vi "Merge in DB.vi"(0 "DBMap in":refnum<class "DBMap.lvclass">, 5 "SQLite DB Path":path, 11 "error in (no error)":errorcluster {"code" format="Error %.0f"}) -> (4 "DBMap out":refnum<class "DBMap.lvclass">, 15 "error out":errorcluster {"code" format="Error %.0f"})   [LabVIEW 2020, in "DBMap.lvclass"]
uses:
  DBMap.lvclass
  DBMap.lvclass/DBMap.ctl
  <vilib>/drjdpowell/SQLite Library/SQL Statement/SQL Statement.lvclass/SQL Statement.ctl
  <vilib>/drjdpowell/SQLite Library/SQL Connection/Connection.lvclass
  <vilib>/drjdpowell/SQLite Library/SQL Statement/SQL Statement.lvclass
  <vilib>/drjdpowell/SQLite Library/Transaction Helpers/Transaction.lvlib
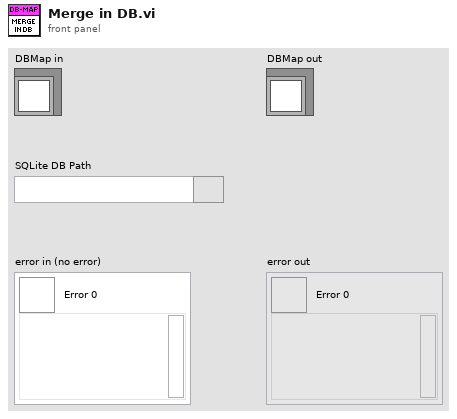
[diagram p1: front panel]
types:
  T1 = typedef "Semaphore RefNum" = refnum<k1>
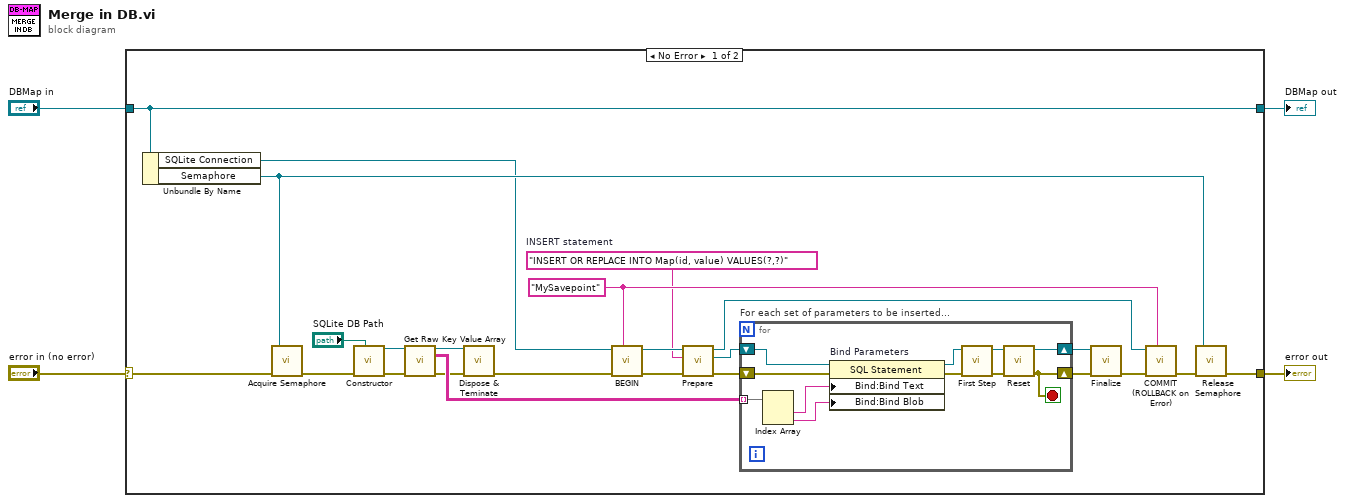
[diagram p0: block diagram]
diagram:
  n1 = case shown="No Error" "error in (no error)" {
    selector: "error in (no error)" -> [w27 w41]
    tunnel: [w26 w41] -> w3
    tunnel: [w28 w40] -> w1
    tunnel: "DBMap in" -> [w28 w40]
    frame No Error {
      w20 = "MySavepoint" ("Savepoint name")
      w15 = "INSERT OR REPLACE INTO Map(id, value) VALUES(?,?)"  # INSERT statement
      n2 = Unbundle By Name(w28) -> ("SQLite Connection"=w8:refnum<class "Connection.lvclass">, "Semaphore"=w25:T1)
      n3 = call <vilib>:"Acquire Semaphore.vi"("error in (no error)"=w27, "semaphore"=w25) -> ("error out"=w24:errorcluster)  [unwired: 3 in, 2 out]
      n4 = call "Constructor.vi"("SQLite DB Path"="SQLite DB Path", "error in (no error)"=w24) -> ("error out"=w11:errorcluster, "DBMap out"=w10:refnum<class "DBMap.lvclass">)  [unwired: 8 in]
      n5 = call "Get Raw Key Value Array.vi"("DBMap in"=w10, "error in (no error)"=w11) -> ("DBMap out"=w5:refnum<class "DBMap.lvclass">, "KV Array Raw"=w9:string[][], "error out"=w7:errorcluster)  [unwired: 11 in]
      n6 = call-dynamic "Dispose & Teminate.vi"("DBMap in"=w5, "error in (no error)"=w7) -> ("error out"=w6:errorcluster)  [unwired: 12 in, 1 out]
      n7 = call <vilib>:"BEGIN.vi"("Savepoint name"=w20, "error in (no error)"=w6, "SQLite Connection in"=w8) -> ("error out"=w19:errorcluster, "SQLite Connection"=w18:refnum<class "Connection.lvclass">)  [unwired: 7 in]
      n8 = call <vilib>:"Prepare.vi"("error in (no error)"=w19, "SQL"=w15, "SQLite Connection in"=w18) -> ("error out"=w14:errorcluster, "SQL Statement"=w13:refnum<class "SQL Statement.lvclass">, "SQLite Connection"=w21:refnum<class "Connection.lvclass">)  [unwired: 4 in, 2 out]
      n9 = for "For each set of parameters to be inserted..." {
        shift-right: [w33] -> w16
        shift-left: w13 -> [w39]
        shift-right: [w32] -> w17
        shift-left: w14 -> [w36]
        tunnel: w9 -> [w31] mode=indexing
        stop <- w32 stop-if-true
        n10 = Index Array(array=w31) -> (element #1=w30:string, element #2=w29:string)  [unwired: 2 in]
        n11 = property on="Bind Parameters" class="SQL Statement"(reference=w39, error in=w36, "Bind:Bind Text"=w30, "Bind:Bind Blob"=w29) -> (reference out=w38:refnum<class "SQL Statement.lvclass">, error out=w37:errorcluster)
        n12 = call <vilib>:"First Step.vi"("error in (no error)"=w37, "SQL Statement in"=w38) -> ("error out"=w35:errorcluster, "SQL Statement"=w34:refnum<class "SQL Statement.lvclass">)  [unwired: 7 in, 1 out]
        n13 = call <vilib>:"Reset.vi"("error in (no error)"=w35, "SQL Statement in"=w34) -> ("error out"=w32:errorcluster, "SQL Statement"=w33:refnum<class "SQL Statement.lvclass">)  [unwired: 8 in]
      }
      n14 = call <vilib>:"Finalize.vi"("error in (no error)"=w17, "SQL Statement in"=w16) -> ("error out"=w22:errorcluster)  [unwired: 9 in]
      n15 = call <vilib>:"COMMIT (ROLLBACK on Error).vi"("Savepoint name"=w20, "error in (no error)"=w22, "SQLite Connection in"=w21) -> ("error out"=w12:errorcluster)  [unwired: 7 in, 1 out]
      n16 = call <vilib>:"Release Semaphore.vi"("error in (no error)"=w12, "semaphore"=w25) -> ("error out"=w26:errorcluster)  [unwired: 4 in, 1 out]
    }
    frame Error {
    }
  }
  "error out" <- w3
  "DBMap out" <- w1
